vi "Waveform Chart Data Types and Update Modes.vi"() -> ()   [LabVIEW 2023]
doc: "This VI illustrates the different kinds of charts and the data types that they can accept. Charts can accept a single point at a time or multiple points at a time. Also, charts can display multiple overlayed or stacked plots. To change between strip, scope, and sweep update modes, right click on the chart and select Advanced->Update Mode."
panel:
  in  "Tab Control":T1(tab)
  out "Single Update (Strip Chart)":dbl(graph)
  out "Single Update (Scope Chart)":dbl(graph)
  out "Single Update (Sweep Chart)":dbl(graph)
  out "Single Update (Multiple Plots)":cluster{dbl, dbl}(graph)
  out "Single Update (Multiple Plots, stacked)":cluster{dbl, dbl}(graph)
  out "Multiple Updates (Single Plot)":dbl[](graph)
  out "Multiple Updates (Multiple Plots)":cluster{dbl, dbl}[](graph)
  in  "Stop":bool
  # "Overview: Demonstrates various waveform chart data types and update modes.\nInstructions:\n1. Run the VI.\n2. Switch between the tabs to observe the appearance of the various waveform charts.\n3. Click Stop to stop the VI."
  # "Single update, single plot waveform charts are scalar data types on the block diagram."
  # "Right-click the chart and select Advanced > Update Mode to choose between Strip Chart, Scope Chart, and Sweep Chart update modes."
  # "Single update, multiple plot waveform charts are cluster data types on the block diagram."
  # "Right-click the chart and select Stack Plots to separate multiple plots into individual plot areas."
  # "Multiple update, single plot waveform charts are array data types on the block diagram. Multiple update, multiple plot waveform charts are array of cluster data types on the block diagram."
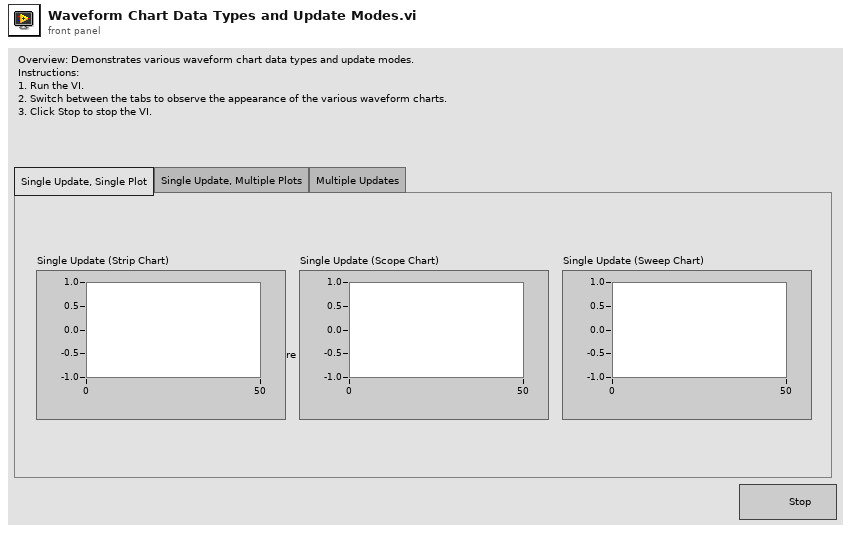
[diagram p1: front panel]
types:
  T1 = enum32{"Single Update, Single Plot", "Single Update, Multiple Plots", "Multiple Updates"}
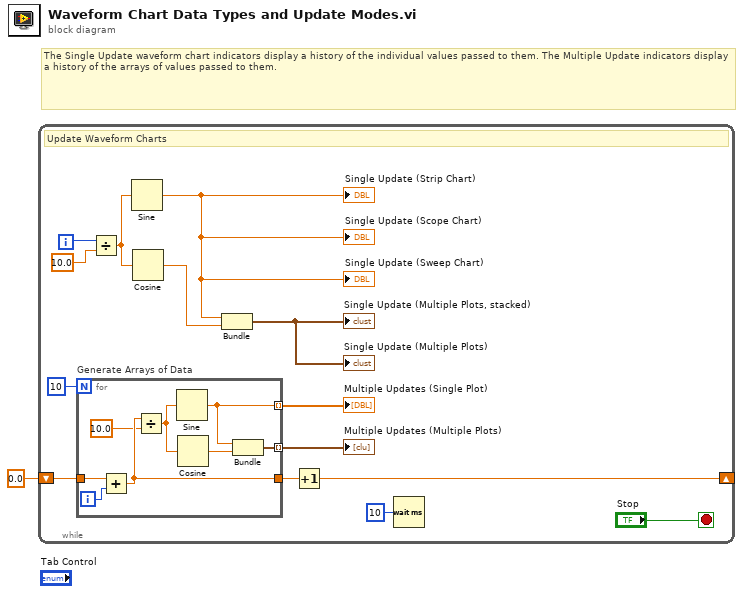
[diagram p0: block diagram]
diagram:
  # "The Single Update waveform chart indicators display a history of the individual values passed to them. The Multiple Update indicators display a history of the arrays of values passed to them."
  n1 = while {
    shift-left: 0.0 -> [w9]
    shift-right: [w8] -> _
    i -> [w15]
    stop <- "Stop" stop-if-true
    # "Update Waveform Charts"
    n2 = for "Generate Arrays of Data" {
      N: 10 ("# of Pts/update") -> [_]
      tunnel: [w22] -> w4 mode=indexing
      tunnel: [w20] -> w3 mode=indexing
      tunnel: [w17] -> w10
      tunnel: w9 -> [w19]
      i -> [w18]
      n3 = Add(x=w19, y=w18) -> (x+y=w17:dbl)
      n4 = Divide(x=w17, y=10.0) -> (x/y=w23:dbl)
      n5 = Sine(x=w23) -> (sin(x)=w22:dbl)
      n6 = Cosine(x=w23) -> (cos(x)=w21:dbl)
      n7 = Bundle(w22, w21) -> (w20:cluster{dbl, dbl})  [unwired: 1 in]
    }
    "Multiple Updates (Multiple Plots)" <- w3
    "Multiple Updates (Single Plot)" <- w4
    n8 = Divide(x=w15, y=10.0) -> (x/y=w14:dbl)
    n9 = Sine(x=w14) -> (sin(x)=w13:dbl)
    "Single Update (Sweep Chart)" <- w13
    "Single Update (Scope Chart)" <- w13
    "Single Update (Strip Chart)" <- w13
    n10 = Cosine(x=w14) -> (cos(x)=w12:dbl)
    n11 = Bundle(w13, w12) -> (→"Single Update (Multiple Plots, stacked)" →"Single Update (Multiple Plots)":cluster{dbl, dbl})  [unwired: 1 in]
    n12 = Increment(x=w10) -> (x+1=w8:dbl)
    n13 = Wait (ms)(milliseconds to wait=u32 10 ("millisecond multiple")) -> ()  [unwired: 1 out]
  }
